vi "Load Config from String.vi"(6 "Fallback Name":string, 8 "error in (no error)":refnum<class "MultiErrors.lvclass">, 10 "JSON":string) -> (0 "error out":refnum<class "MultiErrors.lvclass">, 3 "Sequence Config":refnum<class "Sequence Config.lvclass">)   [LabVIEW 2023, in "VolatusSeqConfig.lvlib" / "Sequence Config.lvclass"]
uses:
  Sequence Config.lvclass
  VolatusErrorUtilities/MultiErrors/MultiErrors.lvclass
  VolatusErrorUtilities/MultiErrors/MultiErrors.lvclass/MultiErrors.ctl
  Sequence Config.lvclass/Sequence Config.ctl
  lv-cdm/CDM-Config/Config-JSON/Config-JSON.lvclass
  lv-cdm/CDM-Config/Config Manager/Config Manager.lvclass
  lv-cdm/CDM-Config/Config Element/Config Element.lvclass
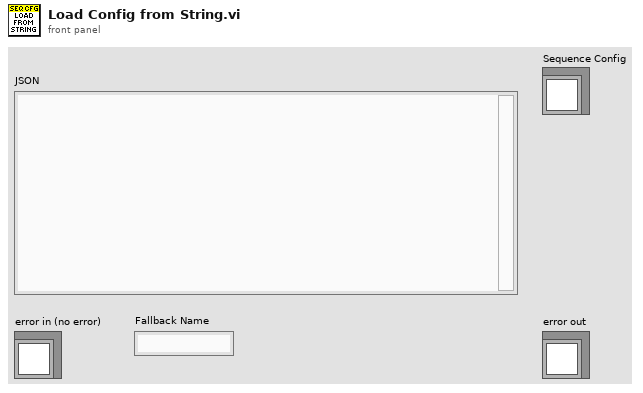
[diagram p1: front panel]
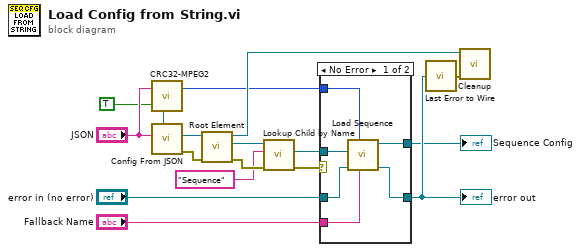
[diagram p0: block diagram]
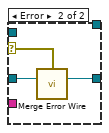
[diagram p2: hidden frame]
diagram:
  n1 = call "CRC32-MPEG2.vi"("Data In"="JSON") -> ("CRC"=w4:u32)  [unwired: 6 in]
  n2 = call "Config From JSON.vi"("Mutable (F)"=TRUE, "JSON"="JSON") -> ("error out"=w10:errorcluster, "Config"=w13:refnum<class "Config Manager.lvclass">)  [unwired: 8 in]
  n3 = call "Root Element.vi"("error in (no error)"=w10, "Config Manager in"=w13) -> ("error out"=w14:errorcluster, "Root Element"=w12:refnum<class "Config Element.lvclass">, "Config Manager out"=w6:refnum<class "Config Manager.lvclass">)  [unwired: 7 in]
  n4 = call "Lookup Child by Name.vi"("error in (no error)"=w14, "Name"="Sequence", "Config Element in"=w12) -> ("error out"=w8:errorcluster, "Child"=w9:refnum<class "Config Element.lvclass">)  [unwired: 5 in, 2 out]
  n5 = case shown="No Error" w8 {
    selector: w8 -> [_ w24]
    tunnel: w9 -> [w22 _]
    tunnel: [w21 _] -> w7
    tunnel: w4 -> [w20 _]
    tunnel: "error in (no error)" -> [w19 w25]
    tunnel: [w18 w23] -> w16
    tunnel: "Fallback Name" -> [w17 _]
    frame No Error {
      n6 = call "Load Sequence.vi"("Fallback Name"=w17, "CRC"=w20, "error in (no error)"=w19, "Config Element"=w22) -> ("error out"=w18:refnum<class "MultiErrors.lvclass">, "Sequence Config out"=w21:refnum<class "Sequence Config.lvclass">)  [unwired: 6 in]
    }
    frame Error {
      n7 = call "Merge Error Wire.vi"("error in (no error)"=w24, "MultiErrors in"=w25) -> ("MultiErrors out"=w23:refnum<class "MultiErrors.lvclass">)  [unwired: 13 in]
    }
  }
  "error out" <- w16
  "Sequence Config" <- w7
  n8 = call "Last Error to Wire.vi"("MultiErrors in"=w16) -> ("error out"=w15:errorcluster)  [unwired: 8 in]
  n9 = call "Cleanup.vi"("error in (no error)"=w15, "Config Manager in"=w6) -> ()  [unwired: 9 in, 1 out]
